vi "Write log file (SubVI).vi"(0 "text":string) -> ()   [LabVIEW 2020]
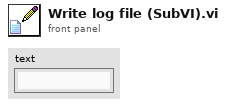
[diagram p1: front panel]
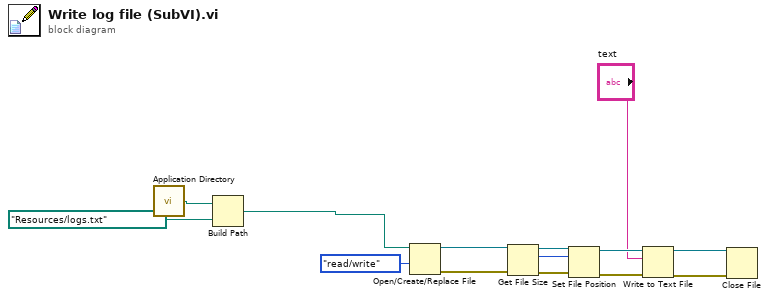
[diagram p0: block diagram]
diagram:
  n1 = call <vilib>:"Application Directory.vi"() -> ("Application Directory"=w13:path)
  n2 = Build Path(base path=w13, name or relative path=path "Resources/logs.txt" ("file path (dialog if empty)")) -> (appended path=w14:path)
  n3 = Open/Create/Replace File(file path (use dialog)=w14, access (0:read/write)=enum16{"read/write", "read-only", "write-only"}."read/write") -> (refnum out=w10:refnum<file>, error out=w9:errorcluster)  [unwired: 4 in, 1 out]
  n4 = Get File Size(file=w10, error in=w9) -> (refnum out=w8:refnum<file>, size (in bytes)=w4:i64, 0:w7:errorcluster)
  n5 = Set File Position(offset (in bytes) (0)=w4, refnum=w8, error in=w7) -> (refnum out=w6:refnum<file>, error out=w5:errorcluster)  [unwired: 1 in]
  n6 = Write to Text File(file (use dialog)=w6, text="text", error in=w5) -> (refnum out=w2:refnum<file>, error out=w1:errorcluster)  [unwired: 1 in, 1 out]
  n7 = Close File(refnum=w2, error in=w1) -> ()  [unwired: 2 out]
